vi "Teleop.vi"(10 "Match Info":T1={"Autonomous Elapsed Seconds"=0.0, "TeleOp Elapsed Seconds"=0.0, "Disabled Elapsed Seconds"=0.0, "Visited Autonomous"=FALSE, "Visited TeleOp"=FALSE, "Visited Disabled"=FALSE, "Autonomous Settings"={"Autonomous Style"=enum."Independent", "VI Refnum"=refnum}}, 11 "Call Context":T2) -> ()   [LabVIEW 2016]
doc: "This VI is called for each enabled TeleOp packet received from the DS. It is typically used to read from joysticks and other inputs and update I/O or setpoints for timed control loops. It should complete and return within 20 milliseconds or risk missing DS packets."
uses:
  <vilib>/Rock Robotics/WPI/DriverStation/WPI_DriverStationDerivedRobotMode.ctl
  <vilib>/Rock Robotics/WPI/DriverStation/WPI_DriverStationMatch Info.ctl
  <vilib>/Rock Robotics/WPI/Solenoid/WPI_SolenoidValue.ctl
  <vilib>/Rock Robotics/WPI/Utilities/WPI_GetSetVariantRefNum.vi
  <vilib>/Rock Robotics/Network Tables/NT Write Boolean Array.vi
  <vilib>/Rock Robotics/Network Tables/NT Write Numeric Array.vi
  <vilib>/Rock Robotics/WPI/Solenoid/Deprecated/WPI_SolenoidGetBool.vi
  <vilib>/Rock Robotics/WPI/RobotDrive/WPI_RobotDriveArcadeDrive_Standard(NoSaturation).vi
  <vilib>/Rock Robotics/WPI/Solenoid/WPI_SolenoidSetEnum.vi
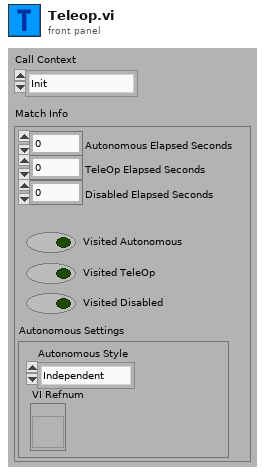
[diagram p1: front panel]
types:
  T1 = typedef "WPI_DriverStationMatch Info.ctl" = cluster{"Autonomous Elapsed Seconds":dbl, "TeleOp Elapsed Seconds":dbl, "Disabled Elapsed Seconds":dbl, "Visited Autonomous":bool, "Visited TeleOp":bool, "Visited Disabled":bool, "Autonomous Settings":cluster{"Autonomous Style":enum16{"Iterative", "Independent"}, "VI Refnum":refnum<vi>}}
  T2 = typedef "WPI_DriverStationDerivedRobotMode.ctl" = enum16{"Init", "Execute", "Stop"}
  T3 = typedef "WPI_SolenoidValue.ctl" = enum16{"Off", "On", "Forward", "Reverse"}
  T4 = typedef "WPI_JoystickDevRef.ctl" = cluster{"Device":T5}
  T5 = typedef "WPI_JoystickDeviceEnum.ctl" = enum16{"USB 0", "USB 1", "USB 2", "USB 3", "USB 4", "USB 5"}
  T6 = cluster{"Axes[0]":dbl, "Axes[1]":dbl, "Axes[2]":dbl, "Axes[3]":dbl, "Axes[4]":dbl, "Axes[5]":dbl, "Axes[6]":dbl, "Axes[7]":dbl, "Axes[8]":dbl}
  T7 = typedef "WPI_RobotDriveDevRef.ctl" = cluster{"DevStatus":errorcluster, "Motors[]":T8[], "Square Inputs":bool, "Max Output":dbl}
  T8 = typedef "WPI_MotorControlDeviceRef.ctl" = cluster{"DeviceStatus":errorcluster, "Type":T9, "PWM":cluster{"PWM Channel":T10, "DeadBand":T11}, "CAN":cluster{"Device Number":u8, "SetOutput VI Ref":variant, "GetOutput VI Ref":variant, "Enable VI Ref":variant, "Disable VI Ref":variant, "Data":variant}, "Invert":bool}
  T9 = typedef "WPI_MotorControlType.ctl" = enum16{"PWM", "CAN"}
  T10 = typedef "FPGA_DIOPWMChannel.ctl" = enum8{"PWM 0", "PWM 1", "PWM 2", "PWM 3", "PWM 4", "PWM 5", "PWM 6", "PWM 7", "PWM 8", "PWM 9", "PWM MXP 0", "PWM MXP 1", "PWM MXP 2", "PWM MXP 3", "PWM MXP 4", "PWM MXP 5", "PWM MXP 6", "PWM MXP 7", "PWM MXP 8", "PWM MXP 9", "Invalid"}
  T11 = typedef "WPI_PWMDeadband.ctl" = cluster{"Name":string, "maxPositivePwm":i32, "minPositivePwm":i32, "centerPwm":i32, "maxNegativePwm":i32, "minNegativePwm":i32, "angularRange":u16}
  T12 = typedef "WPI_SolenoidDevRef.ctl" = cluster{"DevStatus":errorcluster, "Pneumatics Control Module":u8, "Forward Solenoid Channel":T13, "Reverse Solenoid Channel":T13}
  T13 = typedef "WPI_SolenoidChannel.ctl" = enum8{"Solenoid 0", "Solenoid 1", "Solenoid 2", "Solenoid 3", "Solenoid 4", "Solenoid 5", "Solenoid 6", "Solenoid 7", "Invalid"}
  T14 = typedef "WPI_RelayDevRef.ctl" = cluster{"DevStatus":errorcluster, "Relay Channel":T15, "Relay Direction":T16}
  T15 = typedef "FPGA_DIORelayChannel.ctl" = enum8{"Relay 0", "Relay 1", "Relay 2", "Relay 3", "Invalid"}
  T16 = typedef "WPI_RelayDirection.ctl" = enum16{"Both directions", "Forward only", "Reverse only"}
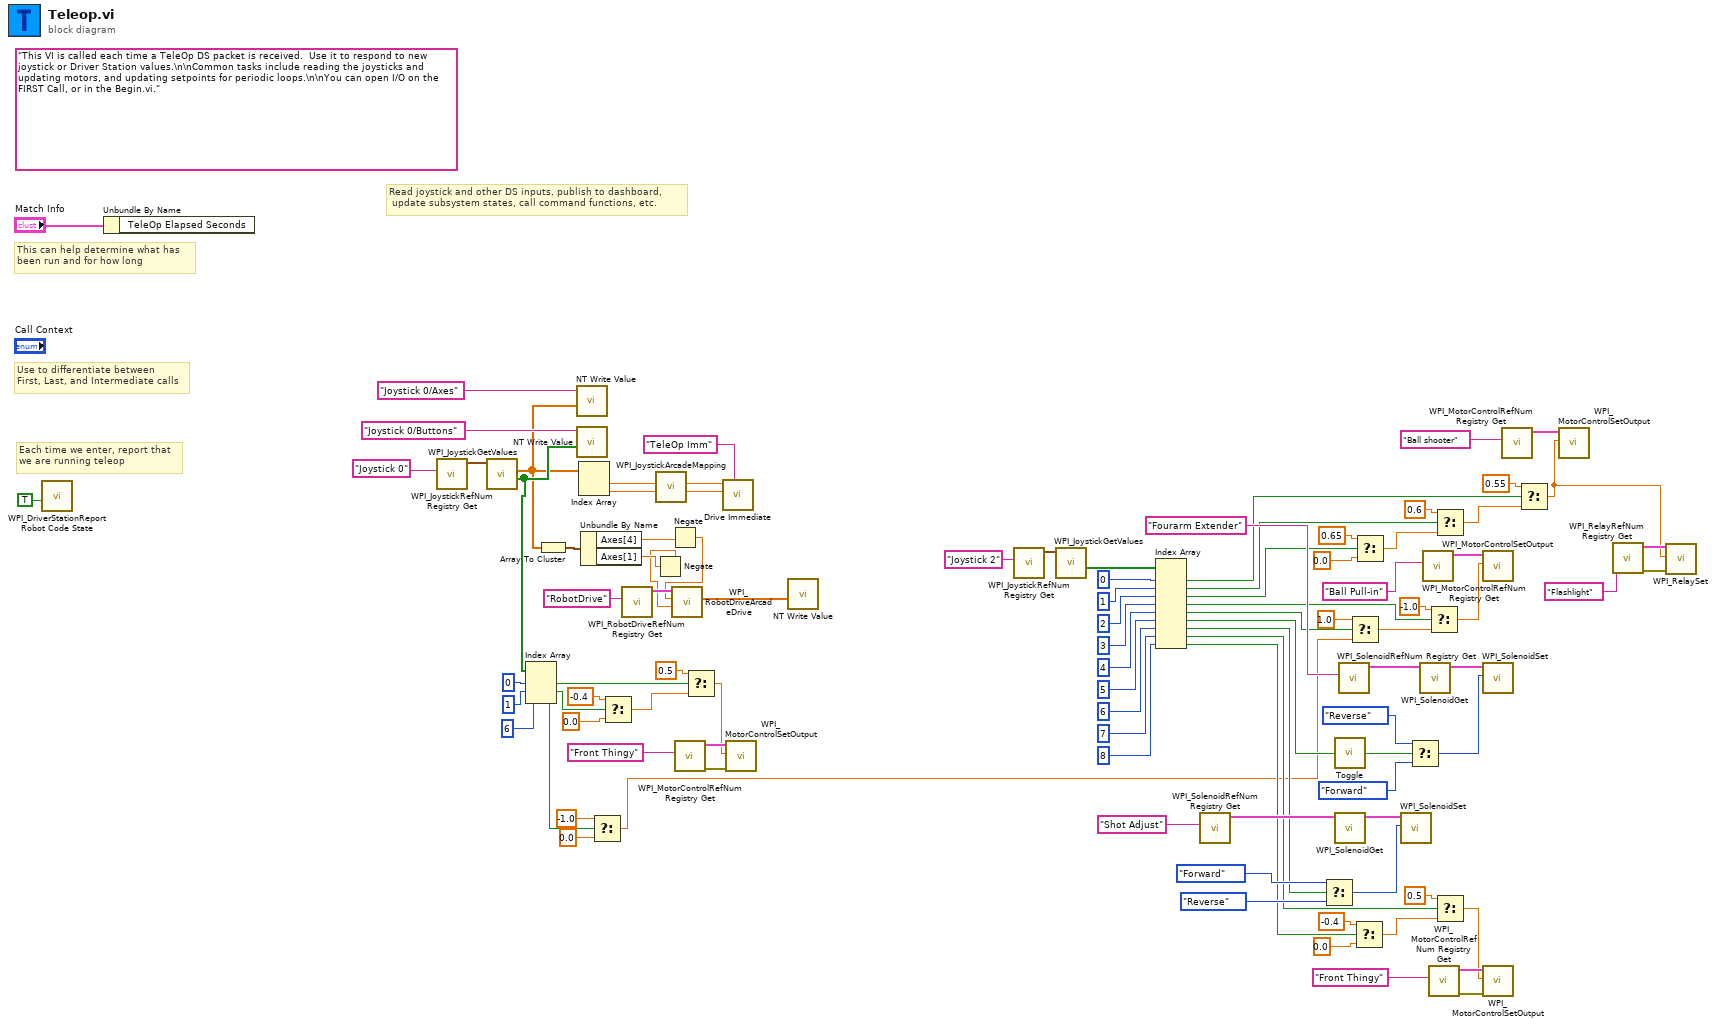
[diagram p0: block diagram]
diagram:
  (unwired) "This VI is called each time a TeleOp DS packet is received.  Use it to respond to new joystick or Driver Station values.\n\nCommon tasks include reading the joysticks and updating motors, and updating setpoints for periodic loops.\n\nYou can open I/O on the FIRST Call, or in the Begin.vi."
  # "Read joystick and other DS inputs, publish to dashboard,\n update subsystem states, call command functions, etc."
  # "Each time we enter, report that\nwe are running teleop"
  # "Use to differentiate between\nFirst, Last, and Intermediate calls"
  # "This can help determine what has\nbeen run and for how long"
  n1 = call <vilib>:"WPI_DriverStationReport Robot Code State.vi"("TeleOp"=TRUE ("Autonomous")) -> ()  [unwired: 10 in, 1 out]
  n2 = Unbundle By Name("Match Info") -> ()  [unwired: 1 out]
  n3 = call <vilib>:"WPI_JoystickRefNum Registry Get.vi"("refnum name"="Joystick 0") -> ("JoystickDevRef"=w95:T4)  [unwired: 1 in, 9 out]
  n4 = call <vilib>:"WPI_JoystickGetValues.vi"("JoystickDevRef"=w95) -> ("Buttons"=w74:bool[], "Axes"=w60:dbl[])  [unwired: 6 in, 3 out]
  n5 = Index Array(array=w74, index #1=0 ("index"), index #2=1 ("index"), index #3=6 ("index")) -> (element #1=w16:bool, element #2=w15:bool, element #3=w12:bool)
  n6 = Array To Cluster(array=w60) -> (cluster=w61:T6)
  n7 = call-poly <vilib>:"NT Write Value.vi"("Numeric Array"=w60, "Name"="Joystick 0/Axes") -> ()  [unwired: 9 in, 1 out]
  n8 = call-poly <vilib>:"NT Write Value.vi"("Boolean Array"=w74, "Name"="Joystick 0/Buttons") -> ()  [unwired: 9 in, 1 out]
  n9 = Index Array(array=w60) -> (element #1=w91:dbl, element #2=w90:dbl)  [unwired: 2 in]
  n10 = Unbundle By Name(w61) -> ("Axes[4]"=w8:dbl, "Axes[1]"=w6:dbl)
  n11 = Select(t=-1.0, s=w12, f=0.0) -> (s? t:f=w9:dbl)
  n12 = Select(t=-0.4, s=w15, f=0.0) -> (s? t:f=w71:dbl)
  n13 = call <vilib>:"WPI_RobotDriveRefNum Registry Get.vi"("refnum name"="RobotDrive" ("Name")) -> ("RobotDriveDevRef"=w64:T7)  [unwired: 9 in, 1 out]
  n14 = Negate(x=w6) -> (-x=w5:dbl)
  n15 = call <vilib>:"WPI_JoystickArcadeMapping.vi"("Y axis value"=w90, "X axis value"=w91) -> ("Right Motor Value"=w92:dbl, "Left Motor Value"=w93:dbl)  [unwired: 8 in]
  n16 = Negate(x=w8) -> (-x=w7:dbl)
  n17 = call-poly <vilib>:"WPI_RobotDriveArcadeDrive.vi"("Y axis value"=w5, "X axis value"=w7, "RobotDriveDevRef"=w64) -> ("Motor Values"=w62:dbl[])  [unwired: 6 in, 2 out]
  n18 = call <vilib>:"WPI_MotorControlRefNum Registry Get.vi"("refnum name"="Front Thingy") -> ("error out"=w66:errorcluster, "MotorControlDevRef"=w67:T8)  [unwired: 9 in]
  n19 = Select(t=0.5, s=w16, f=w71) -> (s? t:f=w65:dbl)
  n20 = call "Drive Immediate.vi"("Description"="TeleOp Imm", "Right Setpoint"=w92, "Left Setpoint"=w93) -> ()  [unwired: 8 in, 1 out]
  n21 = call <vilib>:"WPI_MotorControlSetOutput.vi"("error in (no error)"=w66, "Output"=w65, "MotorControlDevRef"=w67) -> ()  [unwired: 6 in, 3 out]
  n22 = call-poly <vilib>:"NT Write Value.vi"("Numeric Array"=w62) -> ()  [unwired: 10 in, 1 out]
  n23 = call <vilib>:"WPI_JoystickRefNum Registry Get.vi"("refnum name"="Joystick 2") -> ("JoystickDevRef"=w80:T4)  [unwired: 9 in, 1 out]
  n24 = call <vilib>:"WPI_JoystickGetValues.vi"("JoystickDevRef"=w80) -> ("Buttons"=w87:bool[])  [unwired: 6 in, 4 out]
  n25 = Index Array(array=w87, index #1=0 ("index"), index #2=1 ("index"), index #3=2 ("index"), index #4=3 ("index"), index #5=4 ("index"), index #6=5 ("index"), index #7=6 ("index"), index #8=7 ("index"), index #9=8 ("index")) -> (element #1=w56:bool, element #2=w49:bool, element #3=w48:bool, element #4=w45:bool, element #5=w44:bool, element #6=w38:bool, element #7=w27:bool, element #8=w23:bool, element #9=w21:bool)
  n26 = call <vilib>:"WPI_SolenoidRefNum Registry Get.vi"("refnum name"="Shot Adjust") -> ("SolenoidDevRef"=w32:T12)  [unwired: 9 in, 1 out]
  n27 = Select(t=WPI_SolenoidValue."Forward" ("Value"), s=w27, f=WPI_SolenoidValue."Reverse" ("Value")) -> (s? t:f=w26:T3)
  n28 = call "Toggle.vi"("Input"=w38) -> ("Toggled Output"=w37:bool)
  n29 = call-poly <vilib>:"WPI_SolenoidGet.vi"("SolenoidDevRef"=w32) -> ("SolenoidDevRef"=w33:T12)  [unwired: 8 in, 2 out]
  n30 = call <vilib>:"WPI_SolenoidRefNum Registry Get.vi"("refnum name"="Fourarm Extender") -> ("SolenoidDevRef"=w84:T12)  [unwired: 9 in, 1 out]
  n31 = Select(t=1.0, s=w44, f=w9) -> (s? t:f=w42:dbl)
  n32 = Select(t=-0.4, s=w21, f=0.0) -> (s? t:f=w22:dbl)
  n33 = Select(t=0.65, s=w48, f=0.0) -> (s? t:f=w52:dbl)
  n34 = call-poly <vilib>:"WPI_SolenoidSet.vi"("Value"=w26, "SolenoidDevRef"=w33) -> ()  [unwired: 8 in, 2 out]
  n35 = Select(t=WPI_SolenoidValue."Reverse" ("Value"), s=w37, f=WPI_SolenoidValue."Forward" ("Value")) -> (s? t:f=w76:T3)
  n36 = call-poly <vilib>:"WPI_SolenoidGet.vi"("SolenoidDevRef"=w84) -> ("SolenoidDevRef"=w82:T12)  [unwired: 8 in, 2 out]
  n37 = call <vilib>:"WPI_MotorControlRefNum Registry Get.vi"("refnum name"="Ball Pull-in") -> ("MotorControlDevRef"=w46:T8)  [unwired: 9 in, 1 out]
  n38 = Select(t=-1.0, s=w45, f=w42) -> (s? t:f=w41:dbl)
  n39 = call <vilib>:"WPI_MotorControlRefNum Registry Get.vi"("refnum name"="Front Thingy") -> ("error out"=w36:errorcluster, "MotorControlDevRef"=w35:T8)  [unwired: 9 in]
  n40 = Select(t=0.6, s=w49, f=w52) -> (s? t:f=w54:dbl)
  n41 = Select(t=0.5, s=w23, f=w22) -> (s? t:f=w17:dbl)
  n42 = call <vilib>:"WPI_MotorControlSetOutput.vi"("Output"=w41, "MotorControlDevRef"=w46) -> ()  [unwired: 7 in, 3 out]
  n43 = call-poly <vilib>:"WPI_SolenoidSet.vi"("Value"=w76, "SolenoidDevRef"=w82) -> ()  [unwired: 8 in, 2 out]
  n44 = call <vilib>:"WPI_MotorControlSetOutput.vi"("error in (no error)"=w36, "Output"=w17, "MotorControlDevRef"=w35) -> ()  [unwired: 6 in, 3 out]
  n45 = call <vilib>:"WPI_MotorControlRefNum Registry Get.vi"("refnum name"="Ball shooter") -> ("MotorControlDevRef"=w58:T8)  [unwired: 9 in, 1 out]
  n46 = Select(t=0.55, s=w56, f=w54) -> (s? t:f=w2:dbl)
  n47 = call <vilib>:"WPI_MotorControlSetOutput.vi"("Output"=w2, "MotorControlDevRef"=w58) -> ()  [unwired: 7 in, 3 out]
  n48 = call <vilib>:"WPI_RelayRefNum Registry Get.vi"("refnum name"="Flashlight") -> ("error out"=w4:errorcluster, "RelayDevRef"=w3:T14)  [unwired: 9 in]
  n49 = call <vilib>:"WPI_RelaySet.vi"("error in (no error)"=w4, "RelayValue"=w2, "RelayDevRef"=w3) -> ()  [unwired: 7 in, 2 out]
